vi "PMXAdditionalFeaturesDemo.vi"() -> ()   [LabVIEW 2016]
doc: "This VI demonstrates the usage of the additional features of a certain device family (here PMX).\nThese VIs (e.g. ReadParameterSetNumber.vi) are only working for PMX devices and are located within the folder PMX.\n\nIf you try to use one of these VIs with a MGC or with a QuantumX, an error will be thrown."
panel:
  out "DigitalOutBitMask":u16
  out "Device has been connected":bool
  in  "IP address of PMX:":string="172.19.191.225"
  out "DeviceStatus":i32
  out "CurrentParameterSetNumber":i32
  out "Parameter 0 has been loaded":bool
  out "error out":errorcluster caption="Error out"
  # "Please enter the  IP address of your PMX:"
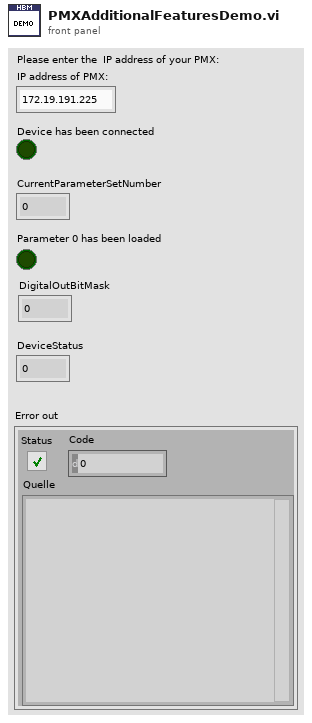
[diagram p1: front panel]
types:
  T1 = cluster{"Devices":refnum<k24>[], "Signals":refnum<k24>[]}
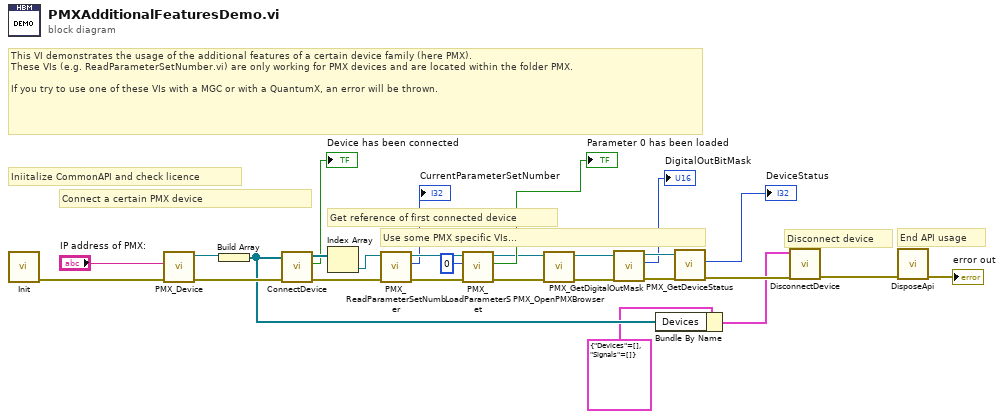
[diagram p0: block diagram]
diagram:
  # "Disconnect device"
  # "End API usage"
  # "Use some PMX specific VIs..."
  # "Get reference of first connected device"
  # "This VI demonstrates the usage of the additional features of a certain device family (here PMX).\nThese VIs (e.g. ReadParameterSetNumber.vi) are only working for PMX devices and are located within the folder PMX.\n\nIf you try to use one of these VIs with a MGC or with a QuantumX, an error will be thrown."
  # "Iniitalize CommonAPI and check licence"
  # "Connect a certain PMX device"
  n1 = call "Init.vi"() -> ("Error out"=w9:errorcluster)  [unwired: 8 in, 2 out]
  n2 = call "PMX_Device.vi"("Error in"=w9, "IPAddress"="IP address of PMX:") -> ("Error out"=w27:errorcluster, "Device"=w14:refnum<k24>)  [unwired: 8 in]
  n3 = Build Array(w14) -> (w3:refnum<k24>[])
  n4 = call "ConnectDevice.vi"("Error in"=w27, "Devices"=w3) -> ("Error out"=w26:errorcluster, "Result"=→"Device has been connected":bool, "Devices"=w13:refnum<k24>[])  [unwired: 7 in]
  n5 = Index Array(array=w13) -> (element=w12:refnum<k24>)  [unwired: 1 in]
  n6 = call "PMX_ReadParameterSetNumber.vi"("Error in"=w26, "Device"=w12) -> ("Error out"=w24:errorcluster, "CurrentParameterSetNumber"=→"CurrentParameterSetNumber":i32, "Device"=w25:refnum<k24>)  [unwired: 7 in]
  n7 = call "PMX_LoadParameterSet.vi"("Error in"=w24, "ParameterSetNumber"=0, "Device"=w25) -> ("Error out"=w15:errorcluster, "Result"=→"Parameter 0 has been loaded":bool, "Device"=w11:refnum<k24>)  [unwired: 6 in]
  n8 = call "PMX_OpenPMXBrowser.vi"("Error in"=w15, "Device"=w11) -> ("Error out"=w20:errorcluster, "Device"=w19:refnum<k24>)  [unwired: 8 in]
  n9 = call "PMX_GetDigitalOutMask.vi"("Error in"=w20, "Device"=w19) -> ("Error out"=w17:errorcluster, "DigitalOutBitMask"=→"DigitalOutBitMask":u16, "Device"=w18:refnum<k24>)  [unwired: 7 in]
  n10 = Bundle By Name(cluster=T1 {"Devices"=[], "Signals"=[]} ("DevicesAndSignals"), "Devices"=w3) -> (w1:T1)
  n11 = call "PMX_GetDeviceStatus.vi"("Error in"=w17, "Device"=w18) -> ("Error out"=w4:errorcluster, "DeviceStatus"=→"DeviceStatus":i32)  [unwired: 7 in, 1 out]
  n12 = call "DisconnectDevice.vi"("Error in"=w4, "DevicesAndSignals"=w1) -> ("Error out"=w5:errorcluster)  [unwired: 9 in]
  n13 = call "DisposeApi.vi"("Error in"=w5) -> ("Error out"=→"error out":errorcluster)  [unwired: 10 in]
